vi "Update-storage-vars.vi"(8 "error in":errorcluster, 11 "Data ref. in":refnum<data-value>) -> (0 "error IO":errorcluster, 3 "Data ref.":refnum<data-value>)   [LabVIEW 2013, in "CameraVision.lvlib" / "CV-Main.lvclass"]
doc: "This function adds a layer/iteration number (-I#) to the base file name, if \"1 file for each layer\" is selected in the storage options. The default storage path construction is '<Storage directory>\\<Base file name>-<Iteration/layer>-<Suffix>-<Index>-<Camera identifier>.<Extension>'."
uses:
  CV-Main.lvclass
  CV-Main.lvclass/CV-Main.ctl
  Read Storage params.vi
  Storage/CV-Storage.lvclass
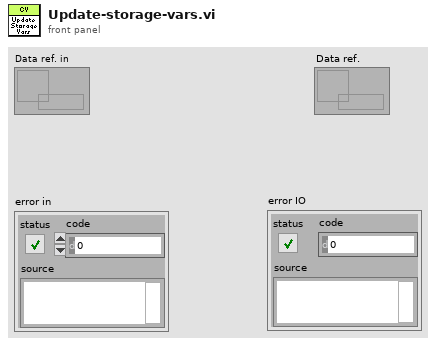
[diagram p1: front panel]
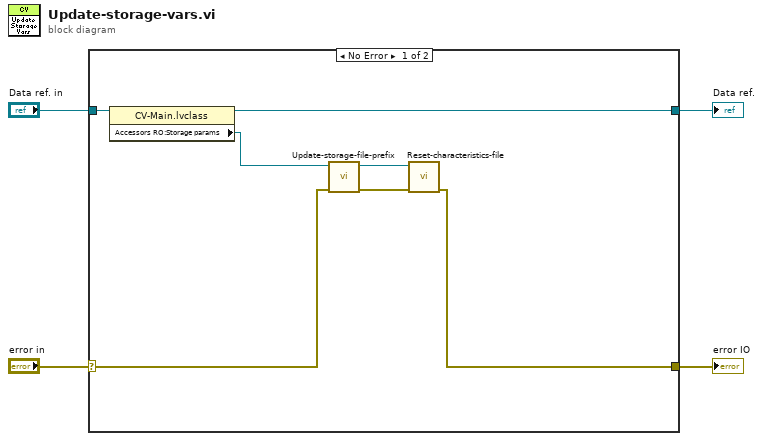
[diagram p0: block diagram]
diagram:
  n1 = case shown="No Error" "error in" {
    selector: "error in" -> [w7 w13]
    tunnel: [w6 w13] -> w3
    tunnel: "Data ref. in" -> [w11 w12]
    tunnel: [w5 w12] -> w1
    frame No Error {
      n2 = property class="CV-Main.lvclass"(reference=w11) -> (reference out=w5:refnum<data-value>, "Accessors RO:Storage params"=w8:refnum<data-value>)  [unwired: 1 in, 1 out]
      n3 = call "Update-storage-file-prefix.vi"("error in (no error)"=w7, "Storage params. ref. in"=w8) -> ("error out"=w9:errorcluster, "Storage params. ref."=w10:refnum<data-value>)  [unwired: 8 in]
      n4 = call "Reset-characteristics-file.vi"("error in (no error)"=w9, "Storage params. ref. in"=w10) -> ("error out"=w6:errorcluster)  [unwired: 8 in, 1 out]
    }
    frame Error {
    }
  }
  "error IO" <- w3
  "Data ref." <- w1
